vi "TestRun.vi"() -> ()   [LabVIEW 2012]
panel:
  in  "Array 3":string[](array[string])=["LOOP.Start(iterations,2)", "Pause(wait.seconds,1)", "LOOP.Start(iterations,3)", "Pause(wait.seconds,2)", "LOOP.End", "LOOP.End", ""]
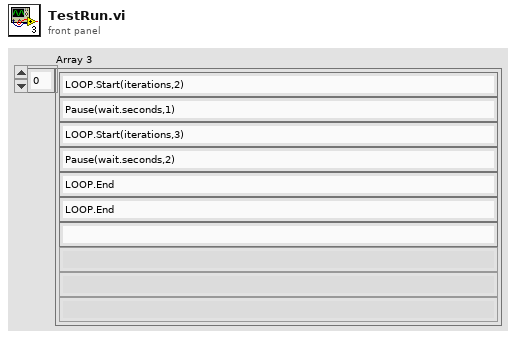
[diagram p1: front panel]
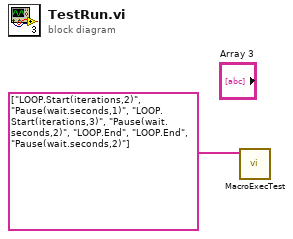
[diagram p0: block diagram]
diagram:
  n1 = call "MacroExecTest.vi"("Macro IN"=string[] ["LOOP.Start(iterations,2)", "Pause(wait.seconds,1)", "LOOP.Start(iterations,3)", "Pause(wait.seconds,2)", "LOOP.End", "LOOP.End", "Pause(wait.seconds,2)"] ("Array 3")) -> ()  [unwired: 10 in, 1 out]
